vi "RestoreDevice.vi"(3 "error in (no error)":errorcluster, 4 "Color modes":u16(ring)=2 items=["RGB"=2, "Y800"=5, "Y16"=11], 5 "Filename":string, 6 "ICImagingControl":refnum<k7>) -> (0 "error out":errorcluster, 1 "IsDeviceValid":bool, 2 "ICImagingControl 2":refnum<k7>)   [LabVIEW 2020]
doc: "This VI is used to open a video capture device. If the specified file does not contain a valid definition, the IC Imaging Control built-in device selection dialog is shown. If a file for device save and restore is specified, the opened video capture device will be saved in this file and opened next time automatically."
uses:
  <vilib>/Utility/error.llb/DialogType.ctl
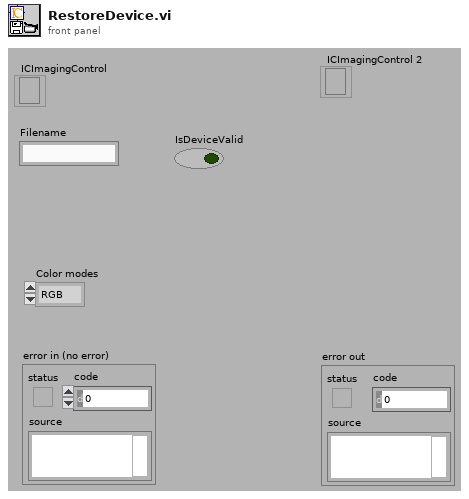
[diagram p1: front panel]
types:
  T1 = typedef "DialogType.ctl" = u16
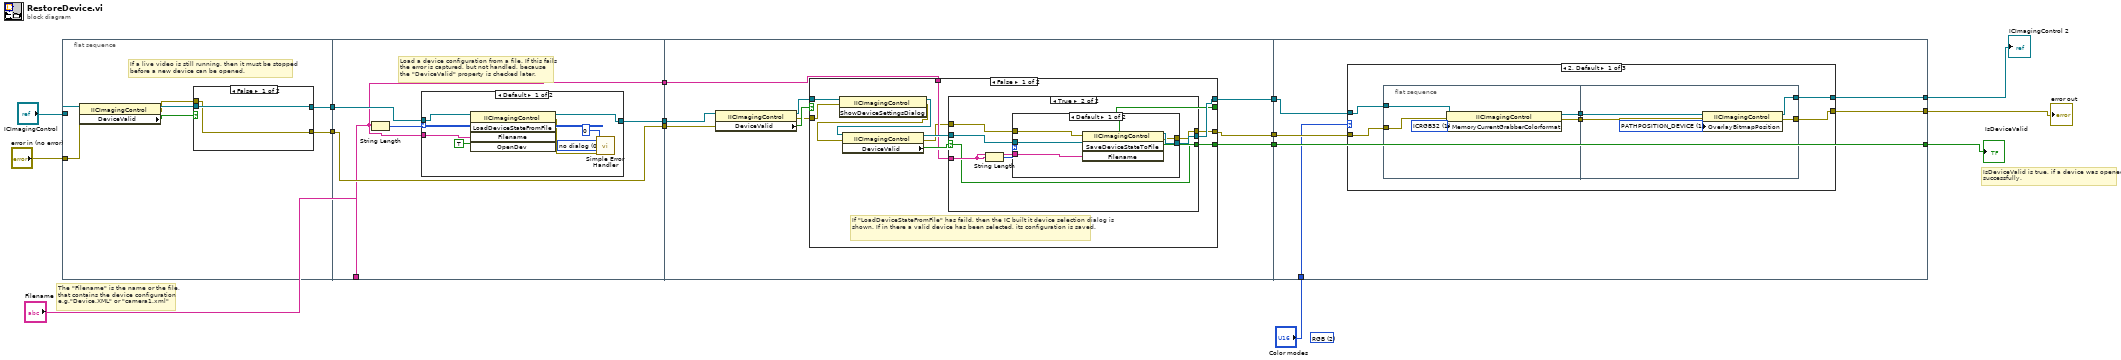
[diagram p0: block diagram]
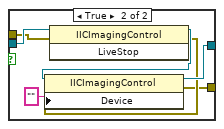
[diagram p2: hidden frame]
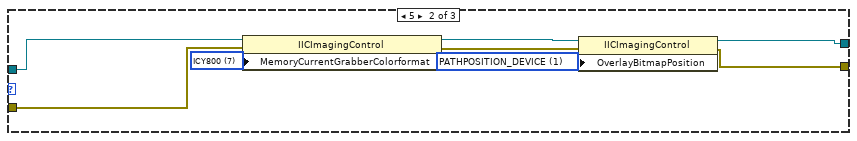
[diagram p7: hidden frame]
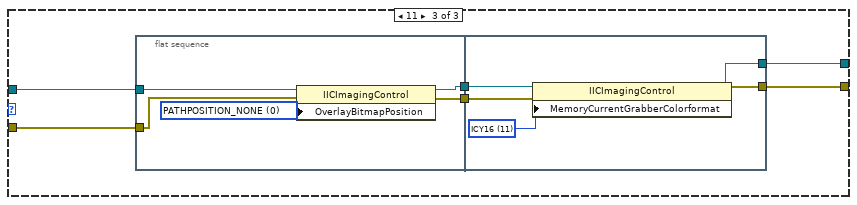
[diagram p8: hidden frame]
diagram:
  (unwired) u16 2 items=["RGB"=2, "Y800"=5, "Y16"=11] ("Color modes")
  # "The \"Filename\" is the name or the file,\nthat contains the device configuration\ne.g.\"Device.XML\" or \"camera1.xml\""
  # "IsDeviceValid is true, if a device was opened\nsuccessfully."
  n1 = flat-sequence {
    tunnel: "ICImagingControl" -> [w22]
    tunnel: "error in (no error)" -> [w19]
    tunnel: [w17] -> w13
    tunnel: [w16] -> w12
    tunnel: w13 -> [w33]
    tunnel: w12 -> [w35]
    tunnel: "Filename" -> [w32]
    tunnel: [w34] -> w10
    tunnel: [w33] -> w9
    tunnel: [w32] -> w8
    tunnel: w10 -> [w53]
    tunnel: w9 -> [w52]
    tunnel: w8 -> [w48]
    tunnel: [w47] -> w7
    tunnel: [w46] -> w6
    tunnel: [w45] -> w5
    tunnel: [w90] -> w4
    tunnel: w7 -> [w90]
    tunnel: w6 -> [w89]
    tunnel: w5 -> [w88]
    tunnel: [w87] -> w3
    tunnel: [w86] -> w2
    tunnel: "Color modes" -> [w85]
    frame #0 {
      # "If a live video is still running, then it must be stopped\nbefore a new device can be opened."
      n2 = property class="IICImagingControl"(reference=w22, error in=w19) -> (reference out=w20:refnum<k7>, error out=w18:errorcluster, "DeviceValid"=w21:bool)
      n3 = case shown="False" w21 {
        tunnel: [w24 w30] -> w16
        tunnel: w20 -> [w24 w28]
        tunnel: w18 -> [w23 w27]
        tunnel: [w23 w25] -> w17
        frame False {
        }
        frame True {
          n4 = invoke class="IICImagingControl" method="LiveStop"(reference=w28, error in=w27) -> (reference out=w31:refnum<k7>, error out=w26:errorcluster)  [unwired: 1 in, 1 out]
          n5 = property class="IICImagingControl"(reference=w31, error in=w26, "Device"="") -> (reference out=w30:refnum<k7>, error out=w25:errorcluster)
        }
      }
    }
    frame #1 {
      # "Load a device configuration from a file. If this fails\nthe error is captured, but not handled, because \nthe \"DeviceValid\" property is checked later."
      n6 = String Length(string=w32) -> (length=w36:i32)
      n7 = case shown="Default" w36 {
        tunnel: w35 -> [w43 w44]
        tunnel: [w42 w44] -> w34
        tunnel: w32 -> [w41 _]
        frame Default {
          w37 = T1 0 items=["no dialog", "OK message", "continue or stop message", "OK message + warnings", "continue/stop + warnings"] ("type of dialog (OK msg:1)")
          n8 = invoke class="IICImagingControl" method="LoadDeviceStateFromFile"(reference=w43, "Filename"=w41, "OpenDev"=TRUE) -> (reference out=w42:refnum<k7>, error out=w39:errorcluster)  [unwired: 2 in, 3 out]
          n9 = call <vilib>:"Simple Error Handler.vi"("error code (no error:0)"=0, "type of dialog (OK msg:1)"=w37, "error in (no error)"=w39) -> ()  [unwired: 2 in, 5 out]
        }
        frame 0 {
        }
      }
    }
    frame #2 {
      n10 = property class="IICImagingControl"(reference=w53, error in=w52) -> (reference out=w51:refnum<k7>, error out=w49:errorcluster, "DeviceValid"=w50:bool)
      n11 = case shown="False" w50 {
        selector: w50 -> [_ w83]
        tunnel: w51 -> [w64 w84]
        tunnel: [w59 w84] -> w46
        tunnel: [w54 w83] -> _
        tunnel: w48 -> [w60 _]
        tunnel: w49 -> [w58 w82]
        tunnel: [w55 w82] -> w45
        tunnel: [w54 w83] -> w47
        frame False {
          # "If \"LoadDeviceStateFromFile\" has faild, then the IC built it device selection dialog is shown. If in there a valid device has been selected, its configuration is saved."
          n12 = invoke class="IICImagingControl" method="ShowDeviceSettingsDialog"(reference=w64, error in=w58) -> (reference out=w63:refnum<k7>, error out=w57:errorcluster)  [unwired: 1 in, 1 out]
          n13 = property class="IICImagingControl"(reference=w63, error in=w57) -> (reference out=w62:refnum<k7>, error out=w56:errorcluster, "DeviceValid"=w61:bool)
          n14 = case shown="True" w61 {
            selector: w61 -> [w66 w68]
            tunnel: w62 -> [w67 w74]
            tunnel: [w67 w71] -> w59
            tunnel: w60 -> [_ w72]
            tunnel: [w66 w68] -> w54
            tunnel: w56 -> [w65 w70]
            tunnel: [w65 w69] -> w55
            frame False {
            }
            frame True {
              n15 = String Length(string=w72) -> (length=w73:i32)
              n16 = case shown="Default" w73 {
                tunnel: w74 -> [w79 w81]
                tunnel: w72 -> [w78 _]
                tunnel: [w77 w81] -> w71
                tunnel: w70 -> [w76 w80]
                tunnel: [w75 w80] -> w69
                frame Default {
                  n17 = invoke class="IICImagingControl" method="SaveDeviceStateToFile"(reference=w79, error in=w76, "Filename"=w78) -> (reference out=w77:refnum<k7>, error out=w75:errorcluster)  [unwired: 1 in, 2 out]
                }
                frame 0 {
                }
              }
            }
          }
        }
        frame True {
          # "LoadDeviceStateFromFile returned a valid device. Thus nothing is to do here."
        }
      }
    }
    frame #3 {
      n18 = case shown="2, Default" w85 {
        tunnel: [w91 w110 w118] -> w87
        tunnel: w89 -> [w96 w109 w117]
        tunnel: w88 -> [w95 w108 w116]
        tunnel: [w93 w107 w115] -> w86
        frame 2, Default {
          n19 = flat-sequence {
            tunnel: w96 -> [w100]
            tunnel: w95 -> [w98]
            tunnel: [w99] -> w94
            tunnel: [w97] -> w92
            tunnel: w94 -> [w105]
            tunnel: [w104] -> w93
            tunnel: w92 -> [w103]
            tunnel: [w102] -> w91
            frame #0 {
              w101 = 1 items=["ICRGB32"=1, "ICRGB24"=2, "ICRGB565"=3, "ICRGB555"=4, "ICY8"=5, "ICUYVY"=6, "ICY800"=7, "ICYGB1"=8, "ICYGB0"=9, "ICBY8"=10, "ICY16"=11] ("MemoryCurrentGrabberColorformat")
              n20 = property class="IICImagingControl"(reference=w100, error in=w98, "MemoryCurrentGrabberColorformat"=w101) -> (reference out=w99:refnum<k7>, error out=w97:errorcluster)
            }
            frame #1 {
              w106 = 1 items=["PATHPOSITION_NONE"=0, "PATHPOSITION_DEVICE"=1, "PATHPOSITION_SINK"=2, "PATHPOSITION_DISPLAY"=4] ("OverlayBitmapPosition")
              n21 = property class="IICImagingControl"(reference=w105, error in=w103, "OverlayBitmapPosition"=w106) -> (reference out=w104:refnum<k7>, error out=w102:errorcluster)
            }
          }
        }
        frame 5 {
          w114 = 1 items=["PATHPOSITION_NONE"=0, "PATHPOSITION_DEVICE"=1, "PATHPOSITION_SINK"=2, "PATHPOSITION_DISPLAY"=4] ("OverlayBitmapPosition")
          w112 = 7 items=["ICRGB32"=1, "ICRGB24"=2, "ICRGB565"=3, "ICRGB555"=4, "ICY8"=5, "ICUYVY"=6, "ICY800"=7, "ICYGB1"=8, "ICYGB0"=9, "ICBY8"=10, "ICY16"=11] ("MemoryCurrentGrabberColorformat")
          n22 = property class="IICImagingControl"(reference=w109, error in=w108, "MemoryCurrentGrabberColorformat"=w112) -> (reference out=w113:refnum<k7>, error out=w111:errorcluster)
          n23 = property class="IICImagingControl"(reference=w113, error in=w111, "OverlayBitmapPosition"=w114) -> (reference out=w107:refnum<k7>, error out=w110:errorcluster)
        }
        frame 11 {
          n24 = flat-sequence {
            tunnel: [w124] -> w120
            tunnel: [w123] -> w119
            tunnel: w117 -> [w122]
            tunnel: w116 -> [w121]
            tunnel: w120 -> [w129]
            tunnel: w119 -> [w128]
            tunnel: [w127] -> w118
            tunnel: [w126] -> w115
            frame #0 {
              w125 = 0 items=["PATHPOSITION_NONE"=0, "PATHPOSITION_DEVICE"=1, "PATHPOSITION_SINK"=2, "PATHPOSITION_DISPLAY"=4] ("OverlayBitmapPosition")
              n25 = property class="IICImagingControl"(reference=w122, error in=w121, "OverlayBitmapPosition"=w125) -> (reference out=w124:refnum<k7>, error out=w123:errorcluster)
            }
            frame #1 {
              w130 = 11 items=["ICRGB32"=1, "ICRGB24"=2, "ICRGB565"=3, "ICRGB555"=4, "ICY8"=5, "ICUYVY"=6, "ICY800"=7, "ICYGB1"=8, "ICYGB0"=9, "ICBY8"=10, "ICY16"=11] ("MemoryCurrentGrabberColorformat")
              n26 = property class="IICImagingControl"(reference=w129, error in=w128, "MemoryCurrentGrabberColorformat"=w130) -> (reference out=w126:refnum<k7>, error out=w127:errorcluster)
            }
          }
        }
      }
    }
  }
  "IsDeviceValid" <- w4
  "error out" <- w3
  "ICImagingControl 2" <- w2
